vi "Generator.AddToQueue.vi"(8 "error in (no error)":errorcluster, 10 "Waveforms":T1, 11 "Generator in":refnum<class "Generator.lvclass">) -> (0 "error out":errorcluster, 3 "Generator out":refnum<class "Generator.lvclass">)   [LabVIEW 2019, in "Generator.lvclass"]
uses:
  Generator.lvclass
  typedefs/Waveforms--Cluster.ctl
  Generator.lvclass/Generator.ctl
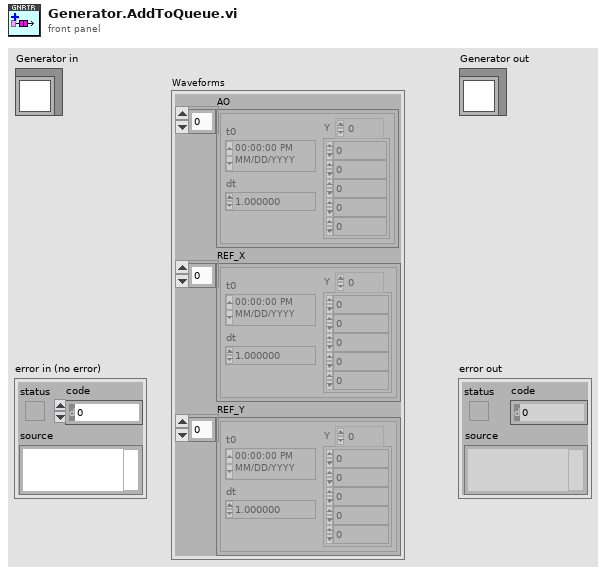
[diagram p1: front panel]
types:
  T1 = typedef "Generator.lvclass/Waveforms--Cluster.ctl" = cluster{"AO":waveform(dbl)[], "REF_X":waveform(dbl)[], "REF_Y":waveform(dbl)[]}
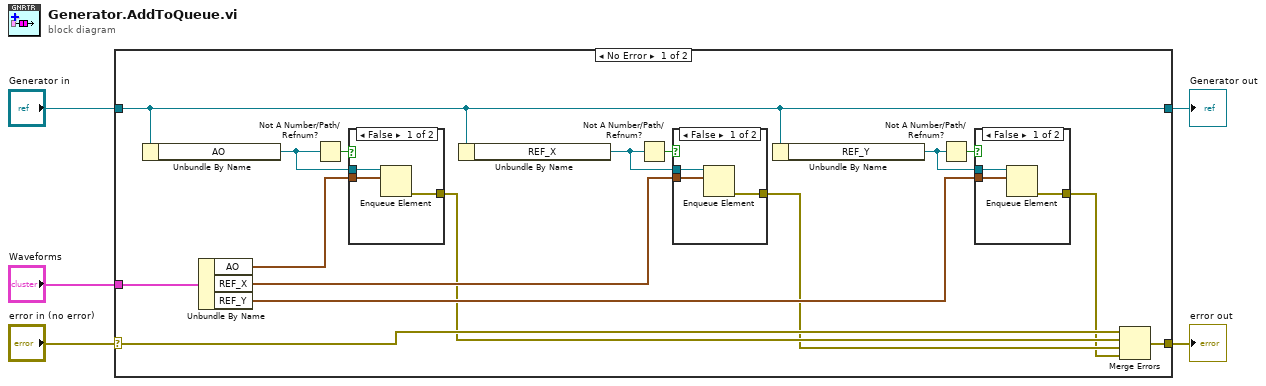
[diagram p0: block diagram]
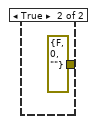
[diagram p2: hidden frame]
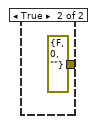
[diagram p3: hidden frame]
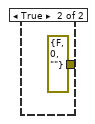
[diagram p4: hidden frame]
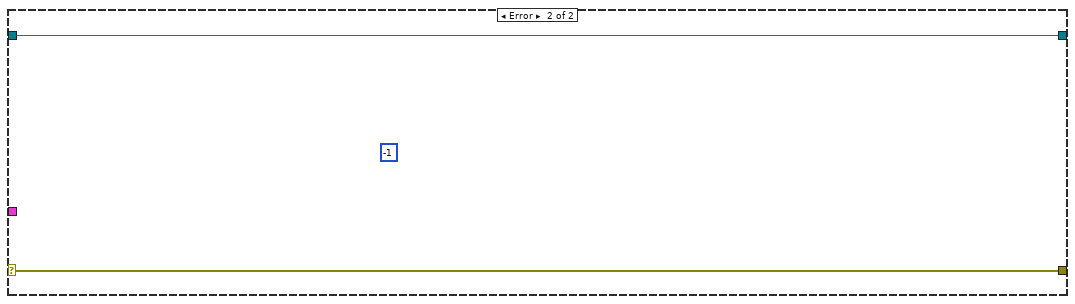
[diagram p5: hidden frame]
diagram:
  n1 = case shown="No Error" "error in (no error)" {
    selector: "error in (no error)" -> [w21 w35]
    tunnel: [w7 w35] -> w4
    tunnel: [w16 w34] -> w2
    tunnel: "Generator in" -> [w16 w34]
    tunnel: "Waveforms" -> [w20 _]
    frame No Error {
      n2 = Unbundle By Name(w16) -> ("AO"=w6:refnum<queue>)
      n3 = Unbundle By Name(w20) -> ("AO"=w19:waveform(dbl)[], "REF_X"=w18:waveform(dbl)[], "REF_Y"=w17:waveform(dbl)[])
      n4 = Not A Number/Path/Refnum?(number/path/refnum=w6) -> (NaN/Path/Refnum?=w15:bool)
      n5 = case shown="False" w15 {
        tunnel: [w24 errorcluster {"status"=FALSE, "code"=0, "source"=""} ("error out")] -> w14
        tunnel: w19 -> [w23 _]
        tunnel: w6 -> [w22 _]
        frame False {
          n6 = Enqueue Element(queue=w22, element=w23) -> (error out=w24:errorcluster)  [unwired: 2 in, 2 out]
        }
        frame True {
        }
      }
      n7 = Unbundle By Name(w16) -> ("REF_X"=w12:refnum<queue>)
      n8 = Not A Number/Path/Refnum?(number/path/refnum=w12) -> (NaN/Path/Refnum?=w9:bool)
      n9 = case shown="False" w9 {
        tunnel: [w28 errorcluster {"status"=FALSE, "code"=0, "source"=""} ("error out")] -> w11
        tunnel: w18 -> [w27 _]
        tunnel: w12 -> [w26 _]
        frame False {
          n10 = Enqueue Element(queue=w26, element=w27) -> (error out=w28:errorcluster)  [unwired: 2 in, 2 out]
        }
        frame True {
        }
      }
      n11 = Unbundle By Name(w16) -> ("REF_Y"=w13:refnum<queue>)
      n12 = Not A Number/Path/Refnum?(number/path/refnum=w13) -> (NaN/Path/Refnum?=w8:bool)
      n13 = case shown="False" w8 {
        tunnel: [w32 errorcluster {"status"=FALSE, "code"=0, "source"=""} ("error out")] -> w10
        tunnel: w17 -> [w31 _]
        tunnel: w13 -> [w30 _]
        frame False {
          n14 = Enqueue Element(queue=w30, element=w31) -> (error out=w32:errorcluster)  [unwired: 2 in, 2 out]
        }
        frame True {
        }
      }
      n15 = Merge Errors(w21, w14, w11, w10) -> (w7:errorcluster)
    }
    frame Error {
      (unwired) -1
    }
  }
  "error out" <- w4
  "Generator out" <- w2
